vi "Update Channel Info.vi"(8 "error in (no error)":errorcluster, 10 "Channel Info":refnum<class "ChannelInfo.lvclass">, 11 "Channel in":refnum<class "Channel.lvclass">) -> (0 "error out":errorcluster, 3 "Channel out":refnum<class "Channel.lvclass">)   [LabVIEW 2015, in "Channel.lvlib" / "Channel.lvclass"]
uses:
  Channel.lvclass
  ChannelInfo.lvclass
  Channel.lvclass/Channel.ctl
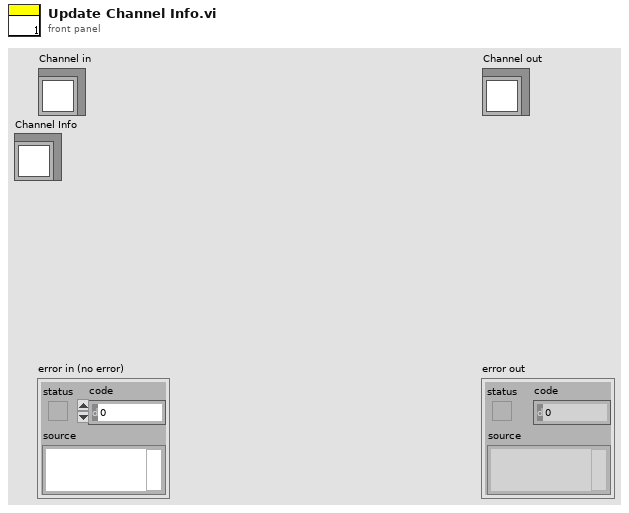
[diagram p1: front panel]
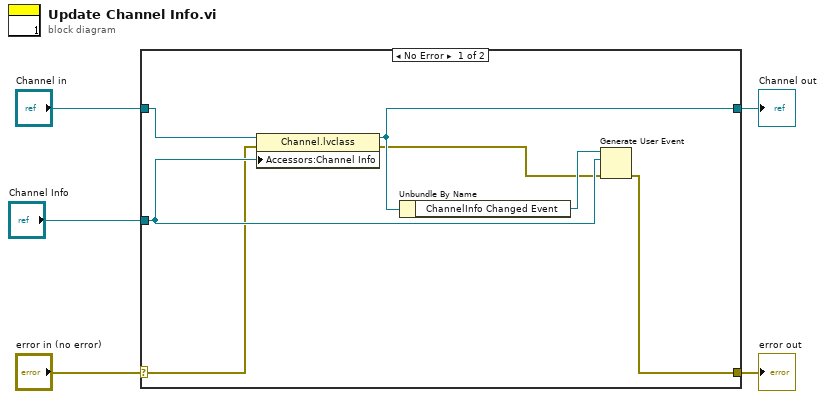
[diagram p0: block diagram]
diagram:
  n1 = case shown="No Error" "error in (no error)" {
    selector: "error in (no error)" -> [w6 w14]
    tunnel: [w7 w14] -> w4
    tunnel: [w11 w13] -> w2
    tunnel: "Channel in" -> [w12 w13]
    tunnel: "Channel Info" -> [w9 _]
    frame No Error {
      n2 = property class="Channel.lvclass"(reference=w12, error in=w6, "Accessors:Channel Info"=w9) -> (reference out=w11:refnum<class "Channel.lvclass">, error out=w8:errorcluster)
      n3 = Unbundle By Name(w11) -> ("ChannelInfo Changed Event"=w10:refnum<user-event>)
      n4 = Generate User Event(user event=w10, event data cluster=w9, error in=w8) -> (error out=w7:errorcluster)  [unwired: 1 in, 1 out]
    }
    frame Error {
    }
  }
  "error out" <- w4
  "Channel out" <- w2
